vi "LobbyBroadcaster.vi"(0 "PlayerInfoMap":T1(c390)) -> ()   [LabVIEW 2025]
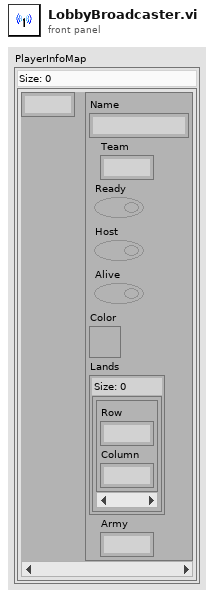
[diagram p1: front panel]
types:
  T1 = map{u32, cluster{"Name":string, "Team":u8, "Ready":bool, "Host":bool, "Alive":bool, "Color":u32, "Lands":set{cluster{"Row":u32, "Column":u32}}, "Army":u32}}
  T2 = cluster{"ID":u32, "Name":string, "Team":u8, "Host":bool, "Ready":bool}[]
  T3 = cluster{"ID":u32, "Name":string, "Team":u8, "Host":bool, "Ready":bool}
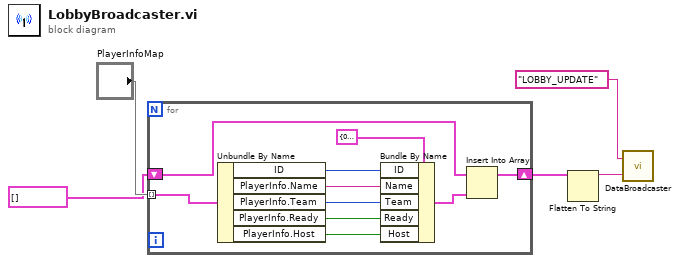
[diagram p0: block diagram]
diagram:
  n1 = for {
    tunnel: "PlayerInfoMap" -> [w14] mode=indexing
    shift-right: [w15] -> w4
    shift-left: T2 [] ("LobbyPlayerInfoArray") -> [w13]
    n2 = Unbundle By Name(w14) -> ("ID"=w11:u32, "PlayerInfo.Name"=w10:string, "PlayerInfo.Team"=w9:u8, "PlayerInfo.Ready"=w8:bool, "PlayerInfo.Host"=w6:bool)
    n3 = Bundle By Name(cluster=T3 {"ID"=0, "Name"="", "Team"=0, "Host"=FALSE, "Ready"=FALSE}, "ID"=w11, "Name"=w10, "Team"=w9, "Ready"=w8, "Host"=w6) -> (w12:T3)
    n4 = Insert Into Array(array=w13, new element=w12) -> (w15:T2)  [unwired: 1 in]
  }
  n5 = Flatten To String(anything=w4) -> (data string=w3:string)  [unwired: 3 in, 2 out]
  n6 = call "DataBroadcaster.vi"("Data"=w3, "Action"="LOBBY_UPDATE") -> ()
